vi "Parse Packet.vi"(11 "data":string) -> (0 "destination address":string, 1 "source address":string, 2 "ip header":T1 {"options / padding" format="%02x"; "fragment offset" format="%04x"; "IHL" format="%02x"; "version" format="%01x"; "type of service" format="%02x"; "total length" format="%02x"; "identification" format="%04x"; "flags" format="%.0x"; "time to live" format="%02x"; "protocol" format="%02.0f"; "header checksum" format="%04x"; "source address" format="%08x"; "destination address" format="%08x"}, 3 "ethernet header":T2 {"destination MAC address"."?" format="%02x"; "destination MAC address"."?" format="%02x"; "destination MAC address"."?" format="%02x"; "destination MAC address"."?" format="%02x"; "destination MAC address"."?" format="%02x"; "destination MAC address"."?" format="%02x"; "source MAC address"."?" format="%02x"; "source MAC address"."?" format="%02x"; "source MAC address"."?" format="%02x"; "source MAC address"."?" format="%02x"; "source MAC address"."?" format="%02x"; "source MAC address"."?" format="%02x"; "length / type" format="%04x"}, 4 "ip data":string, 5 "ip packet":bool)   [LabVIEW 2017]
doc: "This VI parses out the ethernet and IP header from each incoming packet. It does not parse out any TCP or UDP headers. See the block diagram for more information on adding this functionality."
uses:
  control_packet_header_ethernet.ctl
  control_packet_header_ip.ctl
panel:
  # "Select Help»Show Context Help and move the cursor over the VI icon to display help for this VI."
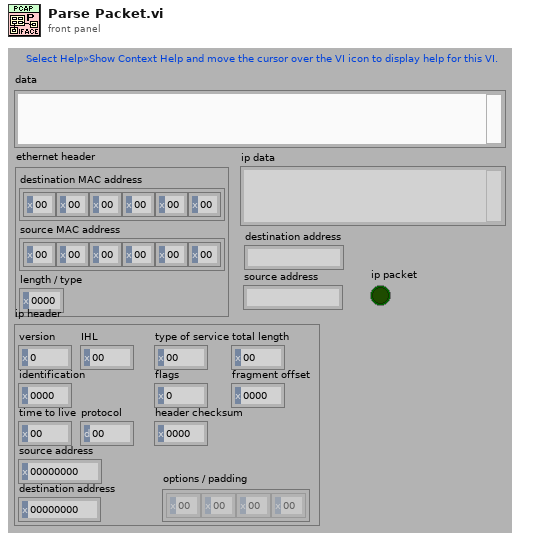
[diagram p1: front panel]
types:
  T1 = typedef "control_packet_header_ip.ctl" = cluster{"version":u8, "IHL":u8, "type of service":u8, "total length":u16, "identification":u16, "flags":u16, "fragment offset":u16, "time to live":u8, "protocol":u8, "header checksum":u16, "source address":u32, "destination address":u32, "options / padding":u8[]}
  T2 = typedef "control_packet_header_ethernet.ctl" = cluster{"destination MAC address":cluster{u8, u8, u8, u8, u8, u8}, "source MAC address":cluster{u8, u8, u8, u8, u8, u8}, "length / type":u16}
  T3 = cluster{"version/IHL":u8, "type of service":u8, "total length":u16, "identification":u16, "flags/fragment offset":u16, "time to live":u8, "protocol":u8, "header checksum":u16, "source address":u32, "destination address":u32}
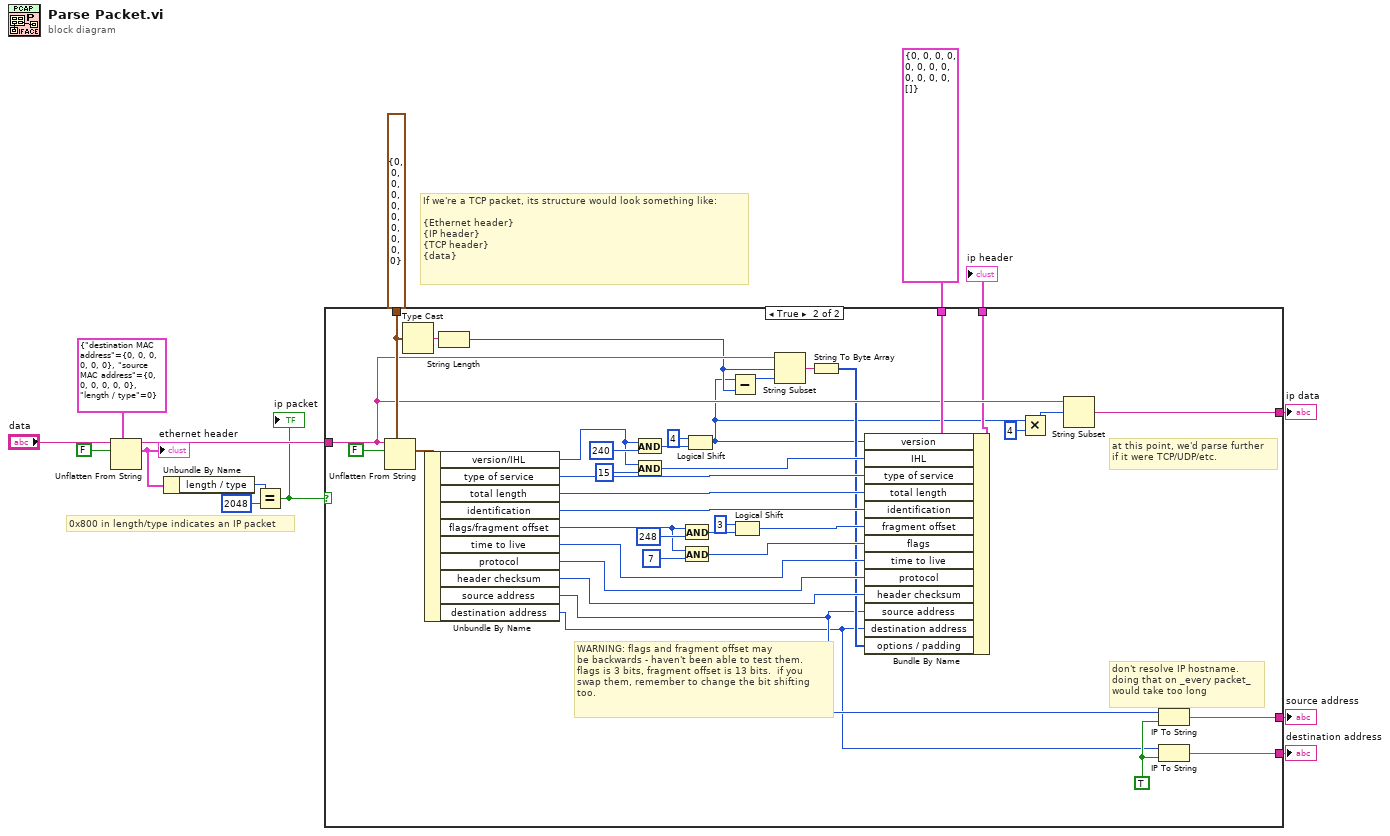
[diagram p0: block diagram]
diagram:
  # "If we're a TCP packet, its structure would look something like:\n\n{Ethernet header}\n{IP header}\n{TCP header}\n{data}"
  # "0x800 in length/type indicates an IP packet"
  n1 = Unflatten From String(type=T2 {"destination MAC address"={0, 0, 0, 0, 0, 0}, "source MAC address"={0, 0, 0, 0, 0, 0}, "length / type"=0} ("ethernet header"), binary string="data", data includes array or string size? (T)=FALSE) -> (rest of the binary string=w8:string, value=w11:T2)  [unwired: 2 in, 1 out]
  "ethernet header" <- w11
  n2 = Unbundle By Name(w11) -> ("length / type"=w10:u16)
  n3 = Equal?(x=w10, y=u16 2048) -> (x = y?=w1:bool)
  "ip packet" <- w1
  n4 = case shown="True" w1 {
    tunnel: w8 -> [_ w23]
    tunnel: T1 {"version"=0, "IHL"=0, "type of service"=0, "total length"=0, "identification"=0, "flags"=0, "fragment offset"=0, "time to live"=0, "protocol"=0, "header checksum"=0, "source address"=0, "destination address"=0, "options / padding"=[]} ("ip header (minus options)") -> [_ w41]
    tunnel: [_ w50] -> w5
    tunnel: [_ w49] -> w4
    tunnel: [_ w48] -> w6
    tunnel: T3 {"version/IHL"=0, "type of service"=0, "total length"=0, "identification"=0, "flags/fragment offset"=0, "time to live"=0, "protocol"=0, "header checksum"=0, "source address"=0, "destination address"=0} ("ip header (minus options)") -> [_ w25]
    tunnel: [_ w18] -> w2
    frame False {
    }
    frame True {
      w47 = TRUE ("dot notation? (F)")
      # "WARNING: flags and fragment offset may\nbe backwards - haven't been able to test them.\nflags is 3 bits, fragment offset is 13 bits.  if you\nswap them, remember to change the bit shifting\ntoo."
      # "at this point, we'd parse further\nif it were TCP/UDP/etc."
      # "don't resolve IP hostname.\ndoing that on _every packet_\nwould take too long"
      n5 = Unflatten From String(type=w25, binary string=w23, data includes array or string size? (T)=FALSE) -> (value=w46:T3)  [unwired: 2 in, 2 out]
      n6 = Type Cast(x=w25) -> (*(type *) &x=w24:string)  [unwired: 1 in]
      n7 = Unbundle By Name(w46) -> ("version/IHL"=w37:u8, "type of service"=w39:u8, "total length"=w38:u16, "identification"=w36:u16, "flags/fragment offset"=w31:u16, "time to live"=w28:u8, "protocol"=w27:u8, "header checksum"=w26:u16, "source address"=w17:u32, "destination address"=w16:u32)
      n8 = String Length(string=w24) -> (length=w22:i32)
      n9 = And(x=w37, y=u8 240) -> (x .and. y?=w43:u8)
      n10 = And(x=w37, y=u8 15) -> (x .and. y?=w40:u8)
      n11 = And(x=w31, y=u8 248) -> (x .and. y?=w34:u16)
      n12 = And(x=w31, y=u8 7) -> (x .and. y?=w29:u16)
      n13 = Logical Shift(y=u8 4, x=w43) -> (x << y=w15:u8)
      n14 = Subtract(x=w15, y=w22) -> (x-y=w21:i32)
      n15 = Logical Shift(y=u8 3, x=w34) -> (x << y=w30:u16)
      n16 = String Subset(string=w23, offset (0)=w22, length (rest)=w21) -> (substring=w20:string)
      n17 = String To Byte Array(string=w20) -> (unsigned byte array=w19:u8[])
      n18 = Bundle By Name(cluster=w41, "version"=w15, "IHL"=w40, "type of service"=w39, "total length"=w38, "identification"=w36, "fragment offset"=w30, "flags"=w29, "time to live"=w28, "protocol"=w27, "header checksum"=w26, "source address"=w17, "destination address"=w16, "options / padding"=w19) -> (w18:T1)
      n19 = Multiply(x=w15, y=u16 4) -> (x*y=w52:u16)
      n20 = String Subset(string=w23, offset (0)=w52) -> (substring=w48:string)  [unwired: 1 in]
      n21 = IP To String(1:w47, 2:w17) -> (0:w50:string)
      n22 = IP To String(1:w47, 2:w16) -> (0:w49:string)
    }
  }
  "ip data" <- w6
  "source address" <- w5
  "destination address" <- w4
  "ip header" <- w2
